vi "Add authenticator to array.vi"(8 "error in (no error)":errorcluster, 10 "IAuthenticator":refnum<class "IAuthenticator.lvclass">, 11 "WAMP Client in":refnum<class "WAMP Client.lvclass">) -> (0 "error out":errorcluster, 3 "WAMP Client out":refnum<class "WAMP Client.lvclass">)   [LabVIEW 2020, in "wamplv.lvlib" / "WAMP Client.lvclass"]
uses:
  WAMP Client.lvclass
  WAMP Client.lvclass/WAMP Client.ctl
  Private/Authenticators/IAuthenticator/IAuthenticator.lvclass
  <vilib>/ErrorRing/Error Ring.xnode
  <vilib>/Utility/error.llb/Error Cluster From Error Code.vi
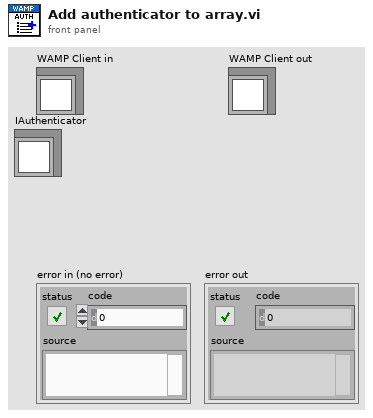
[diagram p1: front panel]
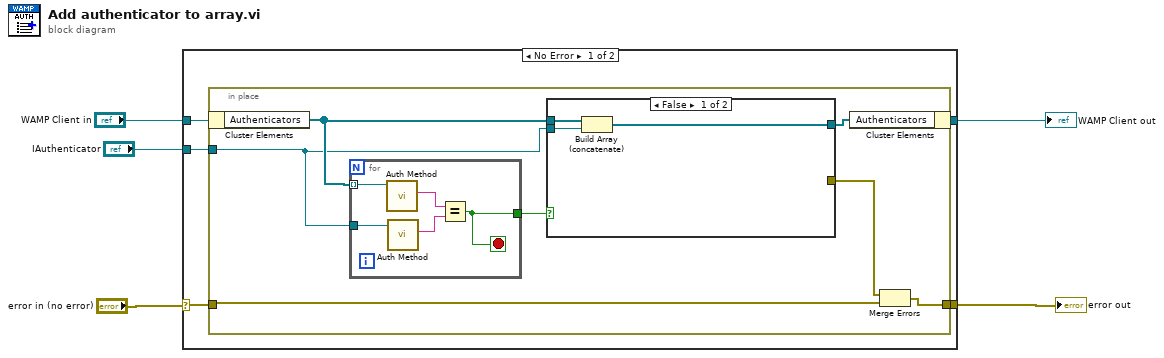
[diagram p0: block diagram]
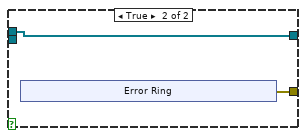
[diagram p2: hidden frame]
diagram:
  n1 = case shown="No Error" "error in (no error)" {
    selector: "error in (no error)" -> [w10 w32]
    tunnel: [w9 w33] -> w4
    tunnel: "WAMP Client in" -> [w8 w33]
    tunnel: [w7 w32] -> w2
    tunnel: "IAuthenticator" -> [w6 _]
    frame No Error {
      n2 = in-place {
        in-place-border: w6 -> [w15]
        in-place-border: w10 -> [w12]
        in-place-border: [w13] -> w7
        n3 = in-place-cluster #1(w8) -> ("Authenticators"=w16:refnum<class "IAuthenticator.lvclass">[])
        n4 = for {
          tunnel: w16 -> [w31] mode=indexing
          tunnel: w15 -> [w30]
          tunnel: [w27] -> w14
          stop <- w27 stop-if-true
          n5 = call-dynamic "Auth Method.vi"("IAuthenticator in"=w31) -> ("Authmethod"=w29:string)  [unwired: 9 in, 1 out]
          n6 = call-dynamic "Auth Method.vi"("IAuthenticator in"=w30) -> ("Authmethod"=w28:string)  [unwired: 9 in, 1 out]
          n7 = Equal?(x=w29, y=w28) -> (x = y?=w27:bool)
        }
        n8 = case shown="False" w14 {
          tunnel: [w20 w22] -> w17
          tunnel: w16 -> [w19 w22]
          tunnel: w15 -> [w18 _]
          tunnel: [_ w21] -> w11
          frame False {
            n9 = Build Array (concatenate)(w19, w18) -> (w20:refnum<class "IAuthenticator.lvclass">[])
          }
          frame True {
            n10 = xnode "Error Ring"() -> ("error out"=w21:errorcluster)
          }
        }
        n11 = in-place-cluster #1("Authenticators"=w17) -> (w9:refnum<class "WAMP Client.lvclass">)
        n12 = Merge Errors(w11, w12) -> (w13:errorcluster)
      }
    }
    frame Error {
    }
  }
  "WAMP Client out" <- w4
  "error out" <- w2
